vi "Phasor Average Lifetime SDV.vi"(0 "tau 1":dbl[unit], 1 "N (1E4)":i32=100000, 5 "tau 2":dbl[unit], 7 "r":dbl, 9 "SDV r":dbl, 11 "Error In":errorcluster, 12 "seed":i32=-1) -> (4 "<tau>_a":dbl[unit] format="%_4f", 6 "SDV <tau>_a":dbl[unit] format="%_4f", 8 "<tau>_i":dbl[unit] format="%_4f", 10 "SDV <tau>_i":dbl[unit] format="%_4f", 14 "SDV a":dbl, 15 "Error Out":errorcluster)   [LabVIEW 2021, in "Phasor.lvlib"]
uses:
  Phasor.lvlib
  <vilib>/gmath/statdist.llb/Normal Random.vi
  <vilib>/gmath/NI_Gmath.lvlib
  <vilib>/Analysis/NI_AALBase.lvlib
  Error/Error.lvlib
  Time/Time.lvlib
panel:
  out "CPU (s)":dbl
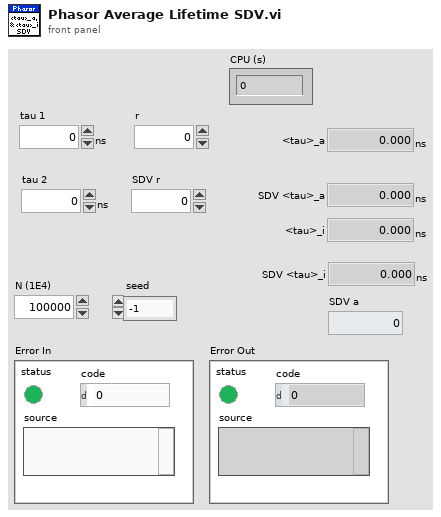
[diagram p1: front panel]
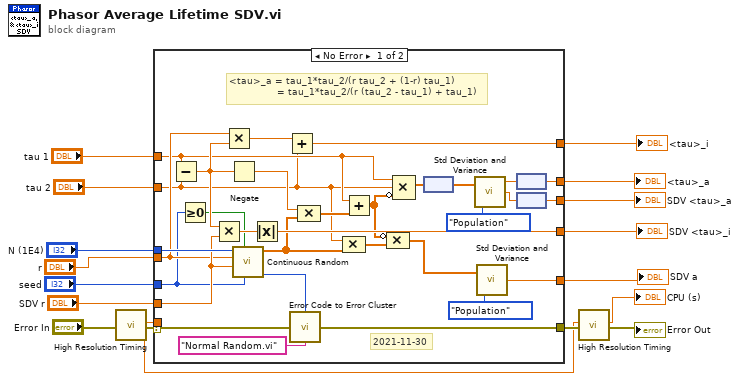
[diagram p0: block diagram]
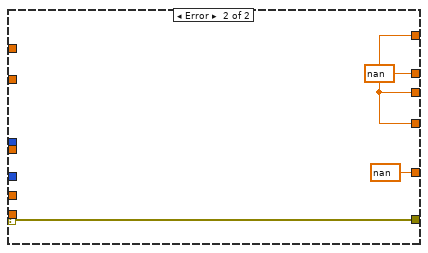
[diagram p2: hidden frame]
diagram:
  n1 = call "High Resolution Timing.vi"("Error In"="Error In") -> ("elapsed (relative) seconds"=w5:dbl, "Error Out"=w9:errorcluster)  [unwired: 16 in, 1 out]
  n2 = case shown="No Error" w9 {
    selector: w9 -> [w40 w51]
    tunnel: "N (1E4)" -> [w48 _]
    tunnel: "r" -> [w33 _]
    tunnel: "SDV r" -> [w36 _]
    tunnel: "tau 2" -> [w25 _]
    tunnel: "tau 1" -> [w28 _]
    tunnel: [w38 w50] -> w12
    tunnel: [w37 w50] -> w11
    tunnel: [w41 w51] -> w10
    tunnel: w5 -> [_ _]
    tunnel: [w34 w50] -> w4
    tunnel: [w31 w50] -> w3
    tunnel: [w26 nan ("mean")] -> w2
    tunnel: "seed" -> [w20 _]
    frame No Error {
      # "2021-11-30"
      # "<tau>_a = tau_1*tau_2/(r tau_2 + (1-r) tau_1)\n                = tau_1*tau_2/(r (tau_2 - tau_1) + tau_1)"
      n3 = Subtract(x=w28, y=w25) -> (x-y=w30:dbl[unit])
      n4 = Greater Or Equal To 0?(x=w20) -> (x >= 0?=w19:bool)
      n5 = Multiply(x=w30, y=w36) -> (x*y=w35:dbl[unit])
      n6 = Multiply(x=w33, y=w30) -> (x*y=w32:dbl[unit])
      n7 = Negate(x=w30) -> (-x=w29:dbl[unit])
      n8 = call-poly <vilib>:"Continuous Random.vi"("seed"=w20, "reset"=w19, "std"=w36, "mean"=w33, "samples"=w48) -> ("error"=w42:i32, "normal random data"=w24:dbl[])  [unwired: 5 in]
      n9 = Absolute Value(x=w35) -> (abs(x)=w34:dbl[unit])
      n10 = Add(x=w32, y=w25) -> (x+y=w31:dbl[unit])
      n11 = call "Error Code to Error Cluster.vi"("Error Code"=w42, "Error Source"="Normal Random.vi", "Error In"=w40) -> ("Error Out"=w41:errorcluster)  [unwired: 12 in]
      n12 = Compound Arithmetic op=MULTIPLY(w29, w24) -> (w47:dbl[unit][])
      n13 = Compound Arithmetic op=MULTIPLY(w25, w24) -> (w23:dbl[unit][])
      n14 = Add(x=w28, y=w47) -> (x+y=w22:dbl[unit][])
      n15 = Compound Arithmetic op=MULTIPLY(invert w22, w23) -> (w21:dbl[])
      n16 = Compound Arithmetic op=MULTIPLY(w28, w25, invert w22) -> (w46:dbl[unit][])
      n17 = node(w46) -> (w39:dbl[])
      n18 = call <vilib>:"Std Deviation and Variance.vi"("X"=w39, "Weighting (Sample)"=enum16{"Sample", "Population"}."Population") -> ("mean"=w44:dbl, "standard deviation"=w43:dbl)  [unwired: 1 out]
      n19 = call <vilib>:"Std Deviation and Variance.vi"("X"=w21, "Weighting (Sample)"=enum16{"Sample", "Population"}."Population") -> ("standard deviation"=w26:dbl)  [unwired: 2 out]
      n20 = node(w44) -> (w38:dbl[unit])
      n21 = node(w43) -> (w37:dbl[unit])
    }
    frame Error {
      w50 = dbl[unit] nan ("mean")
    }
  }
  "<tau>_a" <- w12
  "SDV <tau>_a" <- w11
  "<tau>_i" <- w3
  "SDV <tau>_i" <- w4
  "SDV a" <- w2
  n22 = call "High Resolution Timing.vi"("relative seconds (NaN)"=w5, "Error In"=w10) -> ("elapsed (relative) seconds"=→"CPU (s)":dbl, "Error Out"=→"Error Out":errorcluster)  [unwired: 15 in, 1 out]
